vi "Venta_Producto.vi"(10 "Ingresado":i32, 11 "Venta":T1) -> (1 "Product?":bool, 2 "Mensaje":string, 3 "Feria":i32)   [LabVIEW 2017]
doc: "SubVI utilizado para hacer la venta de producto."
uses:
  Controls/Venta.ctl
  Controls/Data.ctl
  Controls/Data_In.ctl
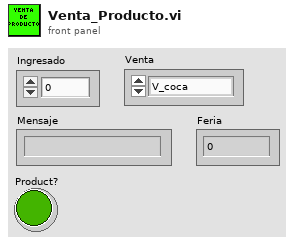
[diagram p1: front panel]
types:
  T1 = typedef "Venta.ctl" = enum16{"V_coca", "V_pepsi"}
  T2 = typedef "Data_In.ctl" = cluster{"Grand Total":i32, "Coca Cola":i32, "Pepsi":i32, "M5":i32, "M2":i32, "M1":i32}
  T3 = typedef "Data.ctl" = enum16{"Grand Total", "Coca-Cola", "Pepsi", "M1", "M2", "M5"}
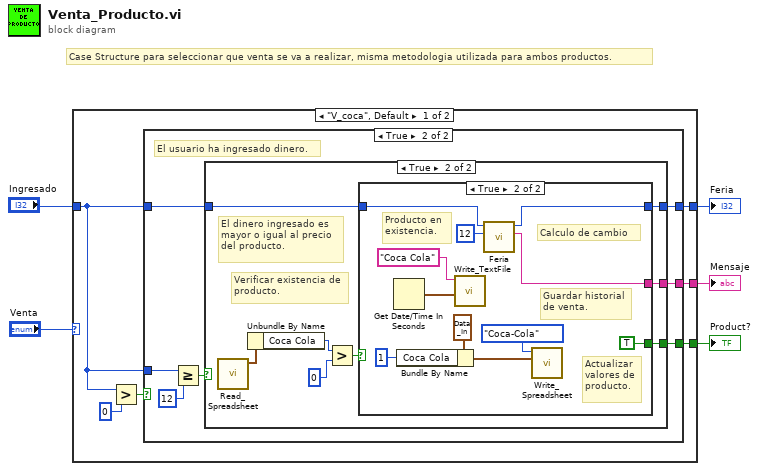
[diagram p0: block diagram]
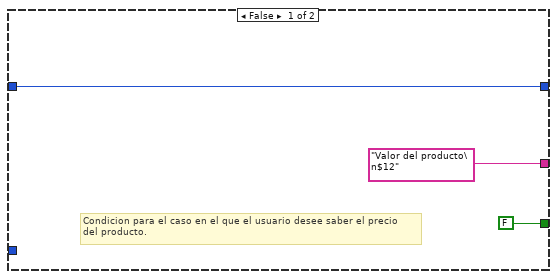
[diagram p2: hidden frame]
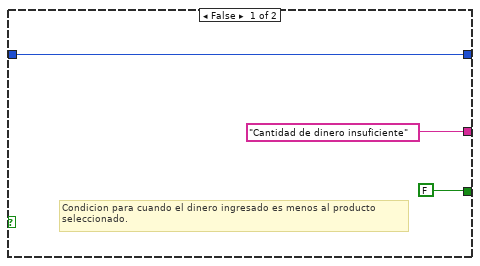
[diagram p3: hidden frame]
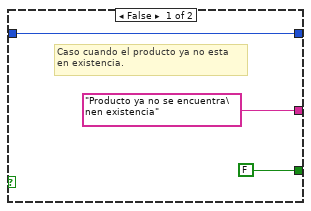
[diagram p4: hidden frame]
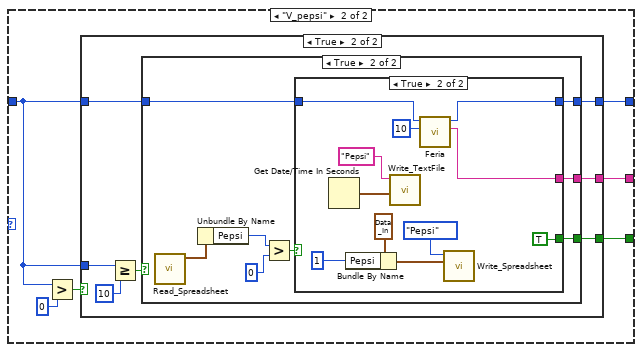
[diagram p5: hidden frame]
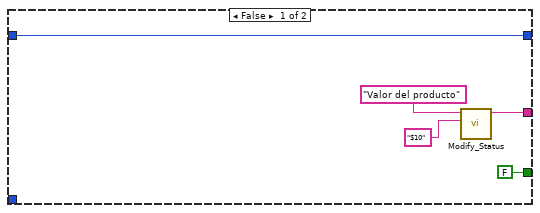
[diagram p6: hidden frame]
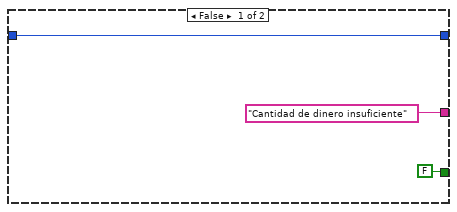
[diagram p7: hidden frame]
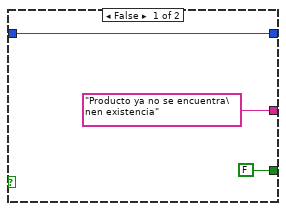
[diagram p8: hidden frame]
diagram:
  # "Case Structure para seleccionar que venta se va a realizar, misma metodologia utilizada para ambos productos."
  n1 = case shown="\"V_coca\", Default" "Venta" {
    tunnel: "Ingresado" -> [w9 w50]
    tunnel: [w8 w49] -> w1
    tunnel: [w7 w48] -> w2
    tunnel: [w6 w47] -> w3
    frame "V_coca", Default {
      n2 = Greater?(x=w9, y=0) -> (0:w10:bool)
      n3 = case shown="True" w10 {
        tunnel: ["Valor del producto\n$12" ("Line 1") w18] -> w7
        tunnel: w9 -> [_ w20]
        tunnel: w9 -> [w14 w17]
        tunnel: [w14 w16] -> w6
        tunnel: [FALSE w15] -> w8
        frame False {
          # "Condicion para el caso en el que el usuario desee saber el precio\ndel producto."
        }
        frame True {
          # "El usuario ha ingresado dinero."
          n4 = Greater Or Equal?(x=w20, y=12) -> (x >= y?=w19:bool)
          n5 = case shown="True" w19 {
            tunnel: ["Cantidad de dinero insuficiente" ("String") w28] -> w18
            tunnel: w17 -> [w23 w27]
            tunnel: [w23 w26] -> w16
            tunnel: [FALSE w25] -> w15
            frame False {
              # "Condicion para cuando el dinero ingresado es menos al producto\nseleccionado."
            }
            frame True {
              # "Verificar existencia de\nproducto."
              # "El dinero ingresado es\nmayor o igual al precio\ndel producto."
              n6 = call "Read_Spreadsheet.vi"() -> ("Data In"=w32:T2)  [unwired: 11 in]
              n7 = Unbundle By Name(w32) -> ("Coca Cola"=w31:i32)
              n8 = Greater?(x=w31, y=0) -> (0:w29:bool)
              n9 = case shown="True" w29 {
                tunnel: ["Producto ya no se encuentra\nen existencia" ("String") w43] -> w28
                tunnel: w27 -> [w34 w46]
                tunnel: [w34 w45] -> w26
                tunnel: [FALSE TRUE] -> w25
                frame False {
                  # "Caso cuando el producto ya no esta\nen existencia."
                }
                frame True {
                  # "Calculo de cambio"
                  # "Guardar historial\nde venta."
                  # "Actualizar \nvalores de\nproducto."
                  # "Producto en\nexistencia."
                  n10 = Get Date/Time In Seconds() -> (seconds since 1Jan1904=w37:timestamp)
                  n11 = Bundle By Name(cluster=T2 {"Grand Total"=0, "Coca Cola"=0, "Pepsi"=0, "M5"=0, "M2"=0, "M1"=0} ("Data In"), "Coca Cola"=1) -> (w40:T2)
                  n12 = call "Write_TextFile.vi"("Fecha"=w37, "Producto"="Coca Cola") -> ()  [unwired: 10 in]
                  n13 = call "Feria.vi"("Precio"=12, "Suma"=w46) -> ("Mensaje"=w43:string, "Feria"=w45:i32)  [unwired: 8 in]
                  n14 = call "Write_Spreadsheet.vi"("Data In"=w40, "Data"=Data."Coca-Cola") -> ()  [unwired: 10 in]
                }
              }
            }
          }
        }
      }
    }
    frame "V_pepsi" {
      n15 = Greater?(x=w50, y=0) -> (0:w51:bool)
      n16 = case shown="True" w51 {
        tunnel: [w55 w61] -> w48
        tunnel: w50 -> [_ w63]
        tunnel: w50 -> [w54 w60]
        tunnel: [w54 w59] -> w47
        tunnel: [FALSE w58] -> w49
        frame False {
          n17 = call "Modify_Status.vi"("Line 2"="$10", "Line 1"="Valor del producto") -> ("resulting string"=w55:string)  [unwired: 9 in]
        }
        frame True {
          n18 = Greater Or Equal?(x=w63, y=10) -> (x >= y?=w62:bool)
          n19 = case shown="True" w62 {
            tunnel: ["Cantidad de dinero insuficiente" ("String") w71] -> w61
            tunnel: w60 -> [w66 w70]
            tunnel: [w66 w69] -> w59
            tunnel: [FALSE w68] -> w58
            frame False {
            }
            frame True {
              n20 = call "Read_Spreadsheet.vi"() -> ("Data In"=w75:T2)  [unwired: 11 in]
              n21 = Unbundle By Name(w75) -> ("Pepsi"=w74:i32)
              n22 = Greater?(x=w74, y=0) -> (0:w72:bool)
              n23 = case shown="True" w72 {
                tunnel: ["Producto ya no se encuentra\nen existencia" ("String") w86] -> w71
                tunnel: w70 -> [w77 w89]
                tunnel: [w77 w88] -> w69
                tunnel: [FALSE TRUE] -> w68
                frame False {
                }
                frame True {
                  n24 = Get Date/Time In Seconds() -> (seconds since 1Jan1904=w80:timestamp)
                  n25 = Bundle By Name(cluster=T2 {"Grand Total"=0, "Coca Cola"=0, "Pepsi"=0, "M5"=0, "M2"=0, "M1"=0} ("Data In"), "Pepsi"=1 ("Coca Cola")) -> (w83:T2)
                  n26 = call "Write_TextFile.vi"("Fecha"=w80, "Producto"="Pepsi") -> ()  [unwired: 10 in]
                  n27 = call "Feria.vi"("Precio"=10, "Suma"=w89) -> ("Mensaje"=w86:string, "Feria"=w88:i32)  [unwired: 8 in]
                  n28 = call "Write_Spreadsheet.vi"("Data In"=w83, "Data"=Data."Pepsi") -> ()  [unwired: 10 in]
                }
              }
            }
          }
        }
      }
    }
  }
  "Feria" <- w3
  "Mensaje" <- w2
  "Product?" <- w1
